vi "get_book_status.vi"(8 "error in (no error)":errorcluster, 11 "librarian in":refnum<class "librarian.lvclass">) -> (0 "error out":errorcluster, 2 "book status":T1, 3 "librarian out":refnum<class "librarian.lvclass">)   [LabVIEW 2020, in "librarian.lvclass"]
uses:
  librarian.lvclass
  typedefs/lib_map_value--cluster.ctl
  typedefs/book_state--enum.ctl
  librarian.lvclass/librarian.ctl
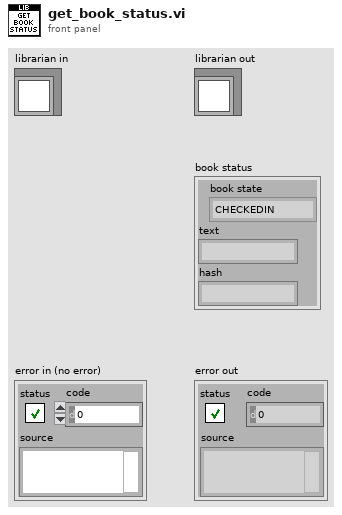
[diagram p1: front panel]
types:
  T1 = typedef "librarian.lvclass/lib_map_value--cluster.ctl" = cluster{"book state":T2, "text":string, "hash":string}
  T2 = typedef "librarian.lvclass/book_state--enum.ctl" = enum16{"CHECKEDIN", "CHECKEDOUT", "DAMAGED"}
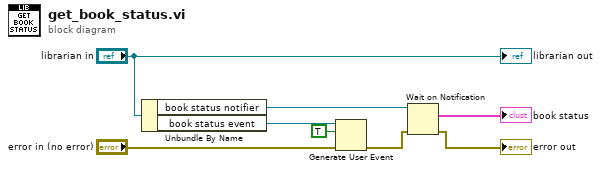
[diagram p0: block diagram]
diagram:
  n1 = Unbundle By Name("librarian in") -> ("book status notifier"=w5:refnum<notifier>, "book status event"=w7:refnum<user-event>)
  n2 = Generate User Event(user event=w7, event data cluster=TRUE ("event data"), error in="error in (no error)") -> (error out=w4:errorcluster)  [unwired: 1 in, 1 out]
  n3 = Wait on Notification(notifier=w5, error in (no error)=w4) -> (notification=→"book status":T1, error out=→"error out":errorcluster)  [unwired: 2 in, 2 out]
  "librarian out" <- "librarian in"
